vi "PID_Controller_Example.vi"() -> ()   [LabVIEW 2019]
uses:
  <vilib>/Rock Robotics/WPI/ThirdParty/JAS_Junk/TrajLib/TypeDef/PID_CONTROLLER.ctl
  <vilib>/Rock Robotics/WPI/ThirdParty/JAS_Junk/TrajLib/SlewRateLimiter_New.vi
  <vilib>/Rock Robotics/WPI/ThirdParty/JAS_Junk/TrajLib/SlewRateLimiter_Reset.vi
  <vilib>/Rock Robotics/WPI/ThirdParty/JAS_Junk/TrajLib/SlewRateLimiter_Calculate.vi
  <vilib>/Rock Robotics/WPI/ThirdParty/JAS_Junk/TrajLib/SlewRateLimiter_SetRate.vi
  <vilib>/Rock Robotics/WPI/ThirdParty/JAS_Junk/TrajLib/PIDController_Calculate_SP_PV.vi
  <vilib>/Rock Robotics/WPI/ThirdParty/JAS_Junk/TrajLib/PIDController_AtSetpoint.vi
  <vilib>/Rock Robotics/WPI/ThirdParty/JAS_Junk/TrajLib/PIDController_SetPID.vi
  <vilib>/Rock Robotics/WPI/ThirdParty/JAS_Junk/TrajLib/PIDController_SetIntegratorRange.vi
  <vilib>/Rock Robotics/WPI/ThirdParty/JAS_Junk/TrajLib/PIDController_SetTolerancePandV.vi
  <vilib>/Rock Robotics/WPI/ThirdParty/JAS_Junk/TrajLib/PIDController_DisableContinousInput.vi
  <vilib>/Rock Robotics/WPI/ThirdParty/JAS_Junk/TrajLib/PIDController_EnableContinousInput.vi
  <vilib>/Rock Robotics/WPI/ThirdParty/JAS_Junk/TrajLib/PIDController_Reset.vi
  <vilib>/Rock Robotics/WPI/ThirdParty/JAS_Junk/TrajLib/PIDController_NewPeriod.vi
  <vilib>/Rock Robotics/WPI/ThirdParty/JAS_Junk/TrajLib/LinearFilter_ResetToValue.vi
  <vilib>/Rock Robotics/WPI/ThirdParty/JAS_Junk/TrajLib/LinearFilter_Calculate.vi
  <vilib>/Rock Robotics/WPI/ThirdParty/JAS_Junk/TrajLib/PIDController_SetSetpoint.vi
  <vilib>/Rock Robotics/WPI/ThirdParty/JAS_Junk/TrajLib/PIDController_Calculate_PV.vi
  <vilib>/Rock Robotics/SystemInterfaces/NetworkCommunication/NetComm_UsageReport_report.vi
  <vilib>/Rock Robotics/WPI/ThirdParty/JAS_Junk/TrajLib/ControllerUtil_GetModulusError.vi
  <vilib>/Rock Robotics/WPI/ThirdParty/JAS_Junk/TrajLib/LinearFilter_MovingAverage.vi
  <vilib>/Rock Robotics/WPI/ThirdParty/JAS_Junk/TrajLib/LinearFilter_LowPassBW1.vi
  <vilib>/Rock Robotics/WPI/ThirdParty/JAS_Junk/TrajLib/LinearFilter_LowPassBW2.vi
  <vilib>/Rock Robotics/WPI/ThirdParty/JAS_Junk/TrajLib/LinearFilter_HighPassBW1.vi
  <vilib>/Rock Robotics/WPI/ThirdParty/JAS_Junk/TrajLib/LinearFilter_HighPassBW2.vi
  <vilib>/Rock Robotics/WPI/ThirdParty/JAS_Junk/TrajLib/Util_LibraryGlobals.vi
  <vilib>/Rock Robotics/WPI/ThirdParty/JAS_Junk/TrajLib/Trajectory_Library.lvlib
panel:
  in  "Tab Control":T1(tab)
  in  "Enable Noise":bool=TRUE
  in  "Auto / Manual":bool=TRUE
  out "Dash Speed Demand":dbl format="%10.2f"
  in  "Desired Speed":dbl(slide)=-0.22222222222222499 scale=-50.0..50.0 scale format="%#.1f"
  out "Dash Speed Target":dbl format="%10.2f"
  out "DashRightMotorOutput":dbl format="%11.3f"
  out "DashRight Wheel Speed":dbl(knob)=-2.895988890827539e-05 scale=-60.0..60.0
  out "Right Wheel ErrorFilt":dbl format="%11.3f"
  out "Right Wheel SpeedFilt":dbl format="%10.2f"
  out "DashLeft Wheel Speed":dbl(knob)=-2.895988890827539e-05 scale=-60.0..60.0
  out "Left Wheel ErrorFilt":dbl format="%11.3f"
  out "DashLeftMotorOutput":dbl format="%11.3f"
  out "Left Wheel Speed Filt":dbl format="%10.2f"
  out "Left CO":dbl format="%13.3f"
  out "Right CO":dbl format="%13.3f"
  out "Duration":dbl format="%11.3f"
  out "Late":dbl format="%11.3f"
  out "SP, PV, CO Left":T2(graph)
  out "SP, PV, CO Right":T2(graph)
  in  "SetPoint Change Rate":dbl=80.0 min=1.0 max=9000.0 format="%14.4f"
  in  "PID Tuning Left":T3={"Kp"=0.4, "Ki"=2.0, "Kd"=0.0, "MaximumIntegral"=1.5, "MinimumIntegral"=-1.5}
  in  "PID Tuning Right":T3={"Kp"=0.4, "Ki"=2.0, "Kd"=0.0, "MaximumIntegral"=1.5, "MinimumIntegral"=-1.5}
  out "Left PID Data":T4={"Kp"=0.0, "Ki"=0.0, "Kd"=0.0, "Period"=0.0, "Max_Integral"=0.0, "Min_Integral"=0.0, "Max_Input"=0.0, "Min_Input"=0.0, "Continuous"=FALSE, "PositionError"=0.0, "VelocityError"=0.0, "PrevError"=0.0, "TotalError"=0.0, "PositionTolerance"=0.0, "VelocityTolerance"=0.0, "SetPoint"=0.0, "Kf"=0.0, "Prev_Deriv"=0.0, "Prev_Deriv 2"=0.0, "DerivativeFilter"=FALSE, "Min_Output"=-9.99e+35, "Max_Output"=9.9e+35, "Prev_F_P"=0.0, "Prev_F_P_2"=0.0, "AntiWindupActive"=FALSE, "Measurement"=0.0} {"Measurement" format="%16_6e"; "Prev_F_P_2" format="%16_6e"; "Prev_F_P" format="%16_6e"; "Max_Output" format="%16_6e"; "Min_Output" format="%16_6e"; "Prev_Deriv 2" format="%16_6e"; "Prev_Deriv" format="%16_6e"; "Kf" format="%16_6e"; "SetPoint" format="%16_6e"; "VelocityTolerance" format="%16_6e"; "PositionTolerance" format="%16_6e"; "TotalError" format="%16_6e"; "PrevError" format="%16_6e"; "VelocityError" format="%16_6e"; "PositionError" format="%16_6e"; "Min_Input" format="%16_6e"; "Max_Input" format="%16_6e"; "Min_Integral" format="%16_6e"; "Max_Integral" format="%16_6e"; "Period" format="%16_6e"; "Kd" format="%16_6e"; "Ki" format="%16_6e"; "Kp" format="%16_6e"}
  out "Right PID Data":T4={"Kp"=0.0, "Ki"=0.0, "Kd"=0.0, "Period"=0.0, "Max_Integral"=0.0, "Min_Integral"=0.0, "Max_Input"=0.0, "Min_Input"=0.0, "Continuous"=FALSE, "PositionError"=0.0, "VelocityError"=0.0, "PrevError"=0.0, "TotalError"=0.0, "PositionTolerance"=0.0, "VelocityTolerance"=0.0, "SetPoint"=0.0, "Kf"=0.0, "Prev_Deriv"=0.0, "Prev_Deriv 2"=0.0, "DerivativeFilter"=FALSE, "Min_Output"=-9.99e+35, "Max_Output"=9.9e+35, "Prev_F_P"=0.0, "Prev_F_P_2"=0.0, "AntiWindupActive"=FALSE, "Measurement"=0.0} {"Measurement" format="%16_6e"; "Prev_F_P_2" format="%16_6e"; "Prev_F_P" format="%16_6e"; "Max_Output" format="%16_6e"; "Min_Output" format="%16_6e"; "Prev_Deriv 2" format="%16_6e"; "Prev_Deriv" format="%16_6e"; "Kf" format="%16_6e"; "SetPoint" format="%16_6e"; "VelocityTolerance" format="%16_6e"; "PositionTolerance" format="%16_6e"; "TotalError" format="%16_6e"; "PrevError" format="%16_6e"; "VelocityError" format="%16_6e"; "PositionError" format="%16_6e"; "Min_Input" format="%16_6e"; "Max_Input" format="%16_6e"; "Min_Integral" format="%16_6e"; "Max_Integral" format="%16_6e"; "Period" format="%16_6e"; "Kd" format="%16_6e"; "Ki" format="%16_6e"; "Kp" format="%16_6e"}
  out "RightWheelSpeed":dbl
  out "LeftWheelSpeed":dbl
  out "RightMotorOutput":dbl
  out "LeftMotorOutput":dbl
  out "SpeedSetpoint":dbl
  in  "SpeedTarget":dbl
  in  "SpeedControlEnabled":bool
  # "PID Controller Example"
  # "This value shows the current speed of each wheel.  This is measured by an encoder.  The encoder measures\n speed by counting pulses of the wheel turning and dividing by the time interval.  Total distance change\nis also a result.  This value is called the \"Process Variable\"."
  # "Enter a desired speed and then press the Set Speed Target \nbutton.  This simulates the joystick input."
  # "FT/SEC"
  # "FT/SEC"
  # "FT/SEC"
  # "FT/SEC"
  # "The Speed Target is rate limited so not to make\nto drastic a change in the desired speed.  (This is\nwhat happens mechanically when pushing the gas\npedal of a real car.)"
  # "This error value shows the error between the current speed\nand the speed demand."
  # "FT/SEC"
  # "This example adds a \"Manual\" mode so that the still operates\nif the encoder fails."
  # "FT/SEC"
  # "FT/SEC"
  # "This value shows the current motor output demand.  This could also be a motor speed demand and \nanother closed loop controller would control the motor speed.  In this simple example this value is \nused to drive the simulated motor directly.  This motor demand is called the \"Control Output\"."
  # "Enables some simulated process noise"
  # "FT/SEC/SEC"
  # "These are the tuning parameters for the PID VI"
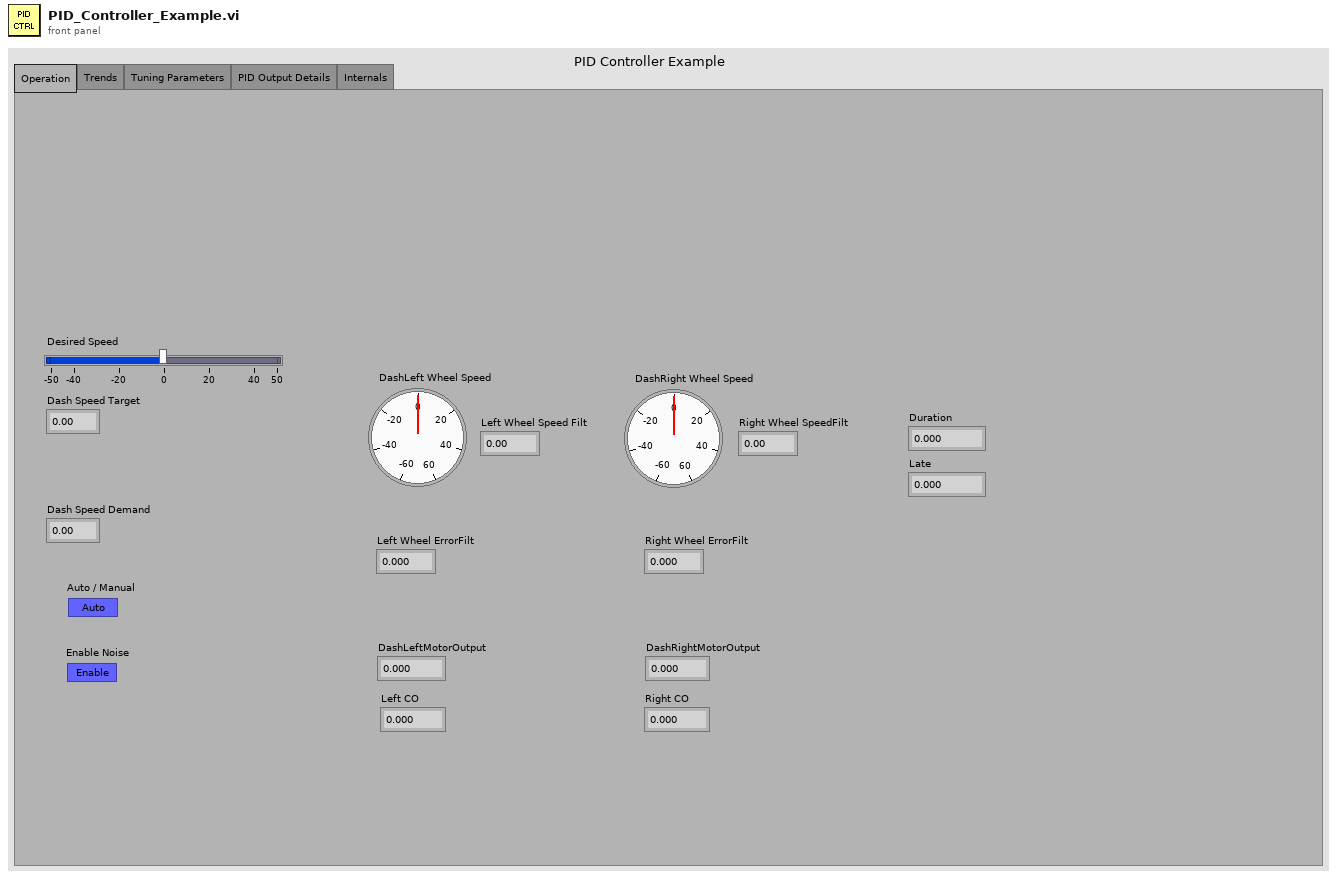
[diagram p1: front panel]
types:
  T1 = enum32{"Operation", "Trends", "Tuning Parameters", "PID Output Details", "Internals"}
  T2 = cluster{"MotorDemand":dbl, "CurrentSetpoint":dbl, "CurrentPosition":dbl}
  T3 = cluster{"Kp":dbl, "Ki":dbl, "Kd":dbl, "MaximumIntegral":dbl, "MinimumIntegral":dbl}
  T4 = typedef "Trajectory_Library.lvlib/PID_CONTROLLER.ctl" = cluster{"Kp":dbl, "Ki":dbl, "Kd":dbl, "Period":dbl, "Max_Integral":dbl, "Min_Integral":dbl, "Max_Input":dbl, "Min_Input":dbl, "Continuous":bool, "PositionError":dbl, "VelocityError":dbl, "PrevError":dbl, "TotalError":dbl, "PositionTolerance":dbl, "VelocityTolerance":dbl, "SetPoint":dbl, "Kf":dbl, "Prev_Deriv":dbl, "Prev_Deriv 2":dbl, "DerivativeFilter":bool, "Min_Output":dbl, "Max_Output":dbl, "Prev_F_P":dbl, "Prev_F_P_2":dbl, "AntiWindupActive":bool, "Measurement":dbl}
  T5 = enum16{"Moving Average", "Low Pass 1st Order Butterworth", "Low Pass 2nd Order Butterworth", "High Pass 1st Order Butterworth", "High Pass 2nd Order Butterworth"}
  T6 = cluster{"LeftMotorOutput":dbl, "SpeedSetpoint":dbl, "LeftWheelSpeed":dbl}
  T7 = cluster{"RightMotorOutput":dbl, "SpeedSetpoint":dbl, "RightWheelSpeed":dbl}
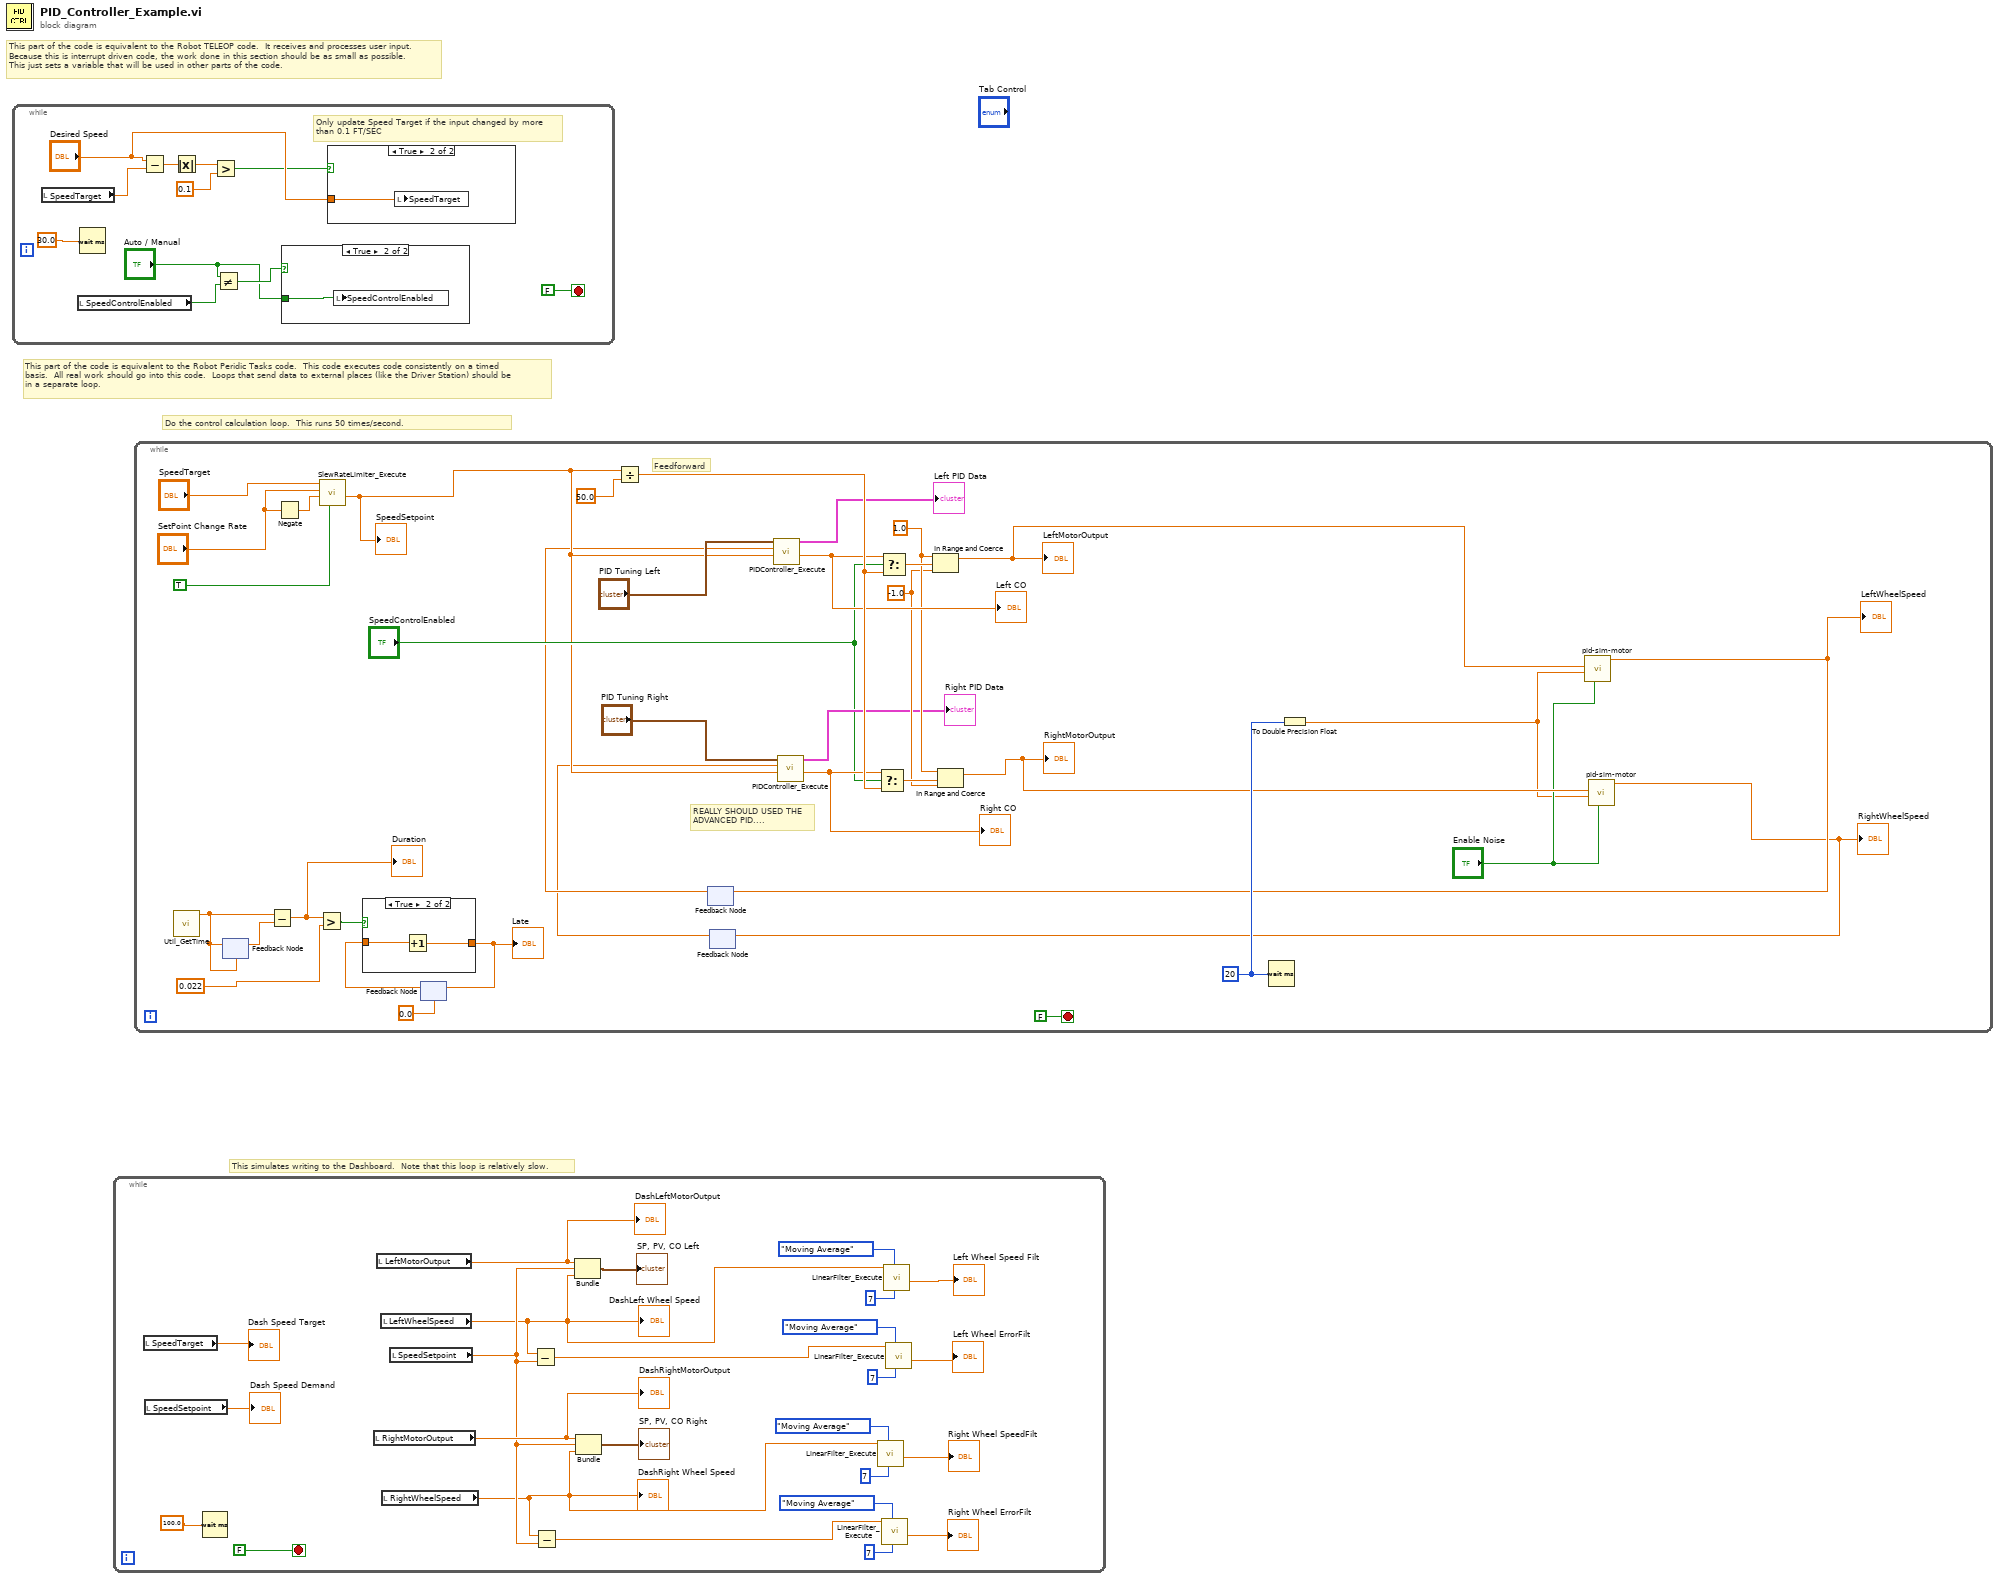
[diagram p0: block diagram]
diagram:
  # "This simulates writing to the Dashboard.  Note that this loop is relatively slow."
  # "Do the control calculation loop.  This runs 50 times/second."
  # "This part of the code is equivalent to the Robot Peridic Tasks code.  This code executes code consistently on a timed\nbasis.  All real work should go into this code.  Loops that send data to external places (like the Driver Station) should be \nin a separate loop."
  # "This part of the code is equivalent to the Robot TELEOP code.  It receives and processes user input.\nBecause this is interrupt driven code, the work done in this section should be as small as possible.\nThis just sets a variable that will be used in other parts of the code."
  n1 = while {
    stop <- FALSE stop-if-true
    # "Only update Speed Target if the input changed by more\nthan 0.1 FT/SEC"
    n2 = local read "SpeedTarget"() -> (w10:dbl)
    n3 = local read "SpeedControlEnabled"() -> (w2:bool)
    n4 = Wait (ms)(milliseconds to wait=30.0) -> ()  [unwired: 1 out]
    n5 = Subtract(x="Desired Speed", y=w10) -> (x-y=w9:dbl)
    n6 = Absolute Value(x=w9) -> (abs(x)=w8:dbl)
    n7 = Greater?(x=w8, y=0.1) -> (0:w5:bool)
    n8 = Not Equal?(x="Auto / Manual", y=w2) -> (x != y?=w3:bool)
    n9 = case shown="True" w3 {
      tunnel: "Auto / Manual" -> [_ w12]
      frame False {
      }
      frame True {
        n10 = local write "SpeedControlEnabled"(w12) -> ()
      }
    }
    n11 = case shown="True" w5 {
      tunnel: "Desired Speed" -> [_ w13]
      frame False {
      }
      frame True {
        n12 = local write "SpeedTarget"(w13) -> ()
      }
    }
  }
  n13 = while {
    stop <- FALSE stop-if-true
    n14 = local read "SpeedTarget"() -> (→"Dash Speed Target":dbl)
    n15 = local read "SpeedSetpoint"() -> (→"Dash Speed Demand":dbl)
    n16 = Wait (ms)(milliseconds to wait=100.0) -> ()  [unwired: 1 out]
    n17 = local read "RightMotorOutput"() -> (w34:dbl)
    "DashRightMotorOutput" <- w34
    n18 = local read "LeftMotorOutput"() -> (w31:dbl)
    "DashLeftMotorOutput" <- w31
    n19 = local read "LeftWheelSpeed"() -> (w27:dbl)
    "DashLeft Wheel Speed" <- w27
    n20 = local read "RightWheelSpeed"() -> (w18:dbl)
    "DashRight Wheel Speed" <- w18
    n21 = local read "SpeedSetpoint"() -> (w30:dbl)
    n22 = Subtract(x=w27, y=w30) -> (x-y=w23:dbl)
    n23 = Subtract(x=w18, y=w30) -> (x-y=w14:dbl)
    n24 = Bundle("LeftMotorOutput"=w31, "SpeedSetpoint"=w30, "LeftWheelSpeed"=w27) -> (→"SP, PV, CO Left":T6)  [unwired: 1 in]
    n25 = Bundle("RightMotorOutput"=w34, "SpeedSetpoint"=w30, "RightWheelSpeed"=w18) -> (→"SP, PV, CO Right":T7)  [unwired: 1 in]
    n26 = call <vilib>:"LinearFilter_Execute.vi"("Samples"=7, "Filter Type"=T5."Moving Average", "Input"=w18) -> ("Output"=→"Right Wheel SpeedFilt":dbl)  [unwired: 7 in, 1 out]
    n27 = call <vilib>:"LinearFilter_Execute.vi"("Samples"=7, "Filter Type"=T5."Moving Average", "Input"=w14) -> ("Output"=→"Right Wheel ErrorFilt":dbl)  [unwired: 7 in, 1 out]
    n28 = call <vilib>:"LinearFilter_Execute.vi"("Samples"=7, "Filter Type"=T5."Moving Average", "Input"=w27) -> ("Output"=→"Left Wheel Speed Filt":dbl)  [unwired: 7 in, 1 out]
    n29 = call <vilib>:"LinearFilter_Execute.vi"("Samples"=7, "Filter Type"=T5."Moving Average", "Input"=w23) -> ("Output"=→"Left Wheel ErrorFilt":dbl)  [unwired: 7 in, 1 out]
  }
  n30 = while {
    stop <- FALSE stop-if-true
    w65 = -1.0 ("lower limit")
    w66 = 1.0 ("upper limit")
    w50 = u32 20 ("milliseconds to wait")
    # "REALLY SHOULD USED THE\nADVANCED PID...."
    # "Feedforward"
    n31 = call <vilib>:"Util_GetTime.vi"() -> ("FPGA_Time_Seconds"=w59:dbl)  [unwired: 10 in, 1 out]
    n32 = feedback #1(w59) -> (w58:dbl)
    n33 = feedback-in #1(w59) -> ()
    n34 = Subtract(x=w59, y=w58) -> (x-y=w56:dbl)
    "Duration" <- w56
    n35 = Negate(x="SetPoint Change Rate") -> (-x=w45:dbl)
    n36 = Greater?(x=w56, y=0.022) -> (0:w57:bool)
    n37 = call <vilib>:"SlewRateLimiter_Execute.vi"("Enable"=TRUE, "NegativeRate"=w45, "PositiveRate"="SetPoint Change Rate", "Input"="SpeedTarget") -> ("Output"=w51:dbl)  [unwired: 6 in, 1 out]
    "SpeedSetpoint" <- w51
    n38 = feedback #2(0.0) -> (w60:dbl)
    n39 = case shown="True" w57 {
      tunnel: [w75 w77] -> w61
      tunnel: w60 -> [w75 w76]
      frame False {
      }
      frame True {
        n40 = Increment(x=w76) -> (x+1=w77:dbl)
      }
    }
    "Late" <- w61
    n41 = feedback-in #2(w61) -> ()
    n42 = Divide(x=w51, y=50.0) -> (x/y=w73:dbl)
    n43 = feedback #3() -> (w49:dbl)  [unwired: 1 in]
    n44 = feedback #4() -> (w48:dbl)  [unwired: 1 in]
    n45 = call <vilib>:"PIDController_Execute.vi"("SP-SetPoint"=w51, "PV-Measurement"=w49, "PID Tuning"="PID Tuning Left") -> ("CO-ControlOutput"=w69:dbl, "out PID_CONTROLLER"=→"Left PID Data":T4)  [unwired: 6 in, 1 out]
    "Left CO" <- w69
    n46 = call <vilib>:"PIDController_Execute.vi"("SP-SetPoint"=w51, "PV-Measurement"=w48, "PID Tuning"="PID Tuning Right") -> ("CO-ControlOutput"=w62:dbl, "out PID_CONTROLLER"=→"Right PID Data":T4)  [unwired: 6 in, 1 out]
    "Right CO" <- w62
    n47 = Select(t=w62, s="SpeedControlEnabled", f=w73) -> (s? t:f=w67:dbl)
    n48 = Select(t=w69, s="SpeedControlEnabled", f=w73) -> (s? t:f=w68:dbl)
    n49 = In Range and Coerce(upper limit=w66, x=w68, lower limit=w65) -> (coerced(x)=w44:dbl)  [unwired: 1 out]
    "LeftMotorOutput" <- w44
    n50 = In Range and Coerce(upper limit=w66, x=w67, lower limit=w65) -> (coerced(x)=w42:dbl)  [unwired: 1 out]
    "RightMotorOutput" <- w42
    n51 = Wait (ms)(milliseconds to wait=w50) -> ()  [unwired: 1 out]
    n52 = To Double Precision Float(number=w50) -> (double precision float=w39:dbl)
    n53 = call "pid-sim-motor.vi"("Use Noise"="Enable Noise", "Cycle Time"=w39, "CO-ControlOutput"=w44) -> ("Motor Speed"=w43:dbl)  [unwired: 8 in]
    "LeftWheelSpeed" <- w43
    n54 = feedback-in #3(w43) -> ()
    n55 = call "pid-sim-motor.vi"("Use Noise"="Enable Noise", "Cycle Time"=w39, "CO-ControlOutput"=w42) -> ("Motor Speed"=w41:dbl)  [unwired: 8 in]
    "RightWheelSpeed" <- w41
    n56 = feedback-in #4(w41) -> ()
  }
